vi "Table Data.vi"() -> ()   [LabVIEW 2018]
panel:
  out "Corner Coordinates":cluster{"X":sgl, "Y":sgl}[](array[cluster])
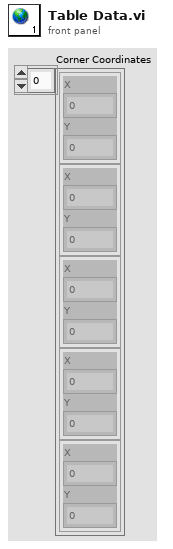
[diagram p1: front panel]
diagram:
